vi "[FPGA] Low Pass Filter Multichannel with Alpha terminal (FXP 16,5).vi"(5 "enable":bool, 7 "Channel #":u32, 10 "LPF alpha":sgl=0.0062437057, 11 "x":sgl) -> (3 "filtered x":sgl)   [LabVIEW 2015]
uses:
  <vilib>/rvi/DataTransferAndStorage/Container/Common/niFpgaContainerGetUniqueNameForEmu.vi
  <vilib>/rvi/DataTransferAndStorage/Container/Common/niFpgaContainerSetEmuInfo.vi
  <vilib>/rvi/eio/common/nirviEmuReportErrorAndStop.vi
  <vilib>/rvi/DataTransferAndStorage/Container/Common/niFpgaContainerExecOnDevCompGetState.vi
  <vilib>/rvi/Emulation/niFpgaEmulationIsFPGAContextNoSignature.vi
  <vilib>/rvi/Emulation/niFpgaProcessEmulError.vi
  <vilib>/rvi/Emulation/niFpgaSctlEmulationGetInTimedLoop.vi
  <vilib>/rvi/errors/nirviReportUnexpectedCaseInternalError (U32).vi
  <vilib>/rvi/Memory/Memory_Emulation/niFpgaMemoryEmulationCacheClearOnFirstRun.vi
  <vilib>/rvi/Memory/Memory_Emulation/nirvimemoryEmulationManagerCache_MakeExclusive.vi
  <vilib>/rvi/Memory/Memory_Emulation/niFpgaMemoryEmulationValidateCache.vi
  <vilib>/rvi/Memory/Memory_Emulation/nirvimemoryEmulationManagerCache_InsertValue.vi
  <vilib>/Utility/error.llb/Clear Errors.vi
  <vilib>/rvi/Memory/Memory_Emulation/nirvimemoryEmulationManagerCache_ReleaseExclusive.vi
  <vilib>/rvi/Memory/Memory_Emulation/nirvimemoryEmulationManagerCache_GetValue.vi
  <vilib>/rvi/Memory/Memory_Emulation/nirvimemoryEmulationManagerCache_SetValue.vi
  <vilib>/rvi/Emulation/niFpgaSctlEmulationResourceMgr.vi
  <vilib>/rvi/LocalResourceManager/LocalResourceManager.xnode
  <vilib>/rvi/DataTransferAndStorage/Container/XNode/niFpgaContainer.xnode
  <vilib>/rvi/Memory/Memory_Emulation/niFpgaMemoryEmulationRefIn.vi
panel:
  # "= 1-1/(2*dT*fc*pi+1)"
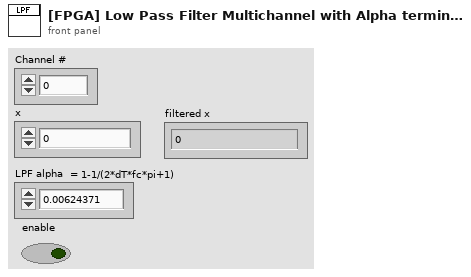
[diagram p1: front panel]
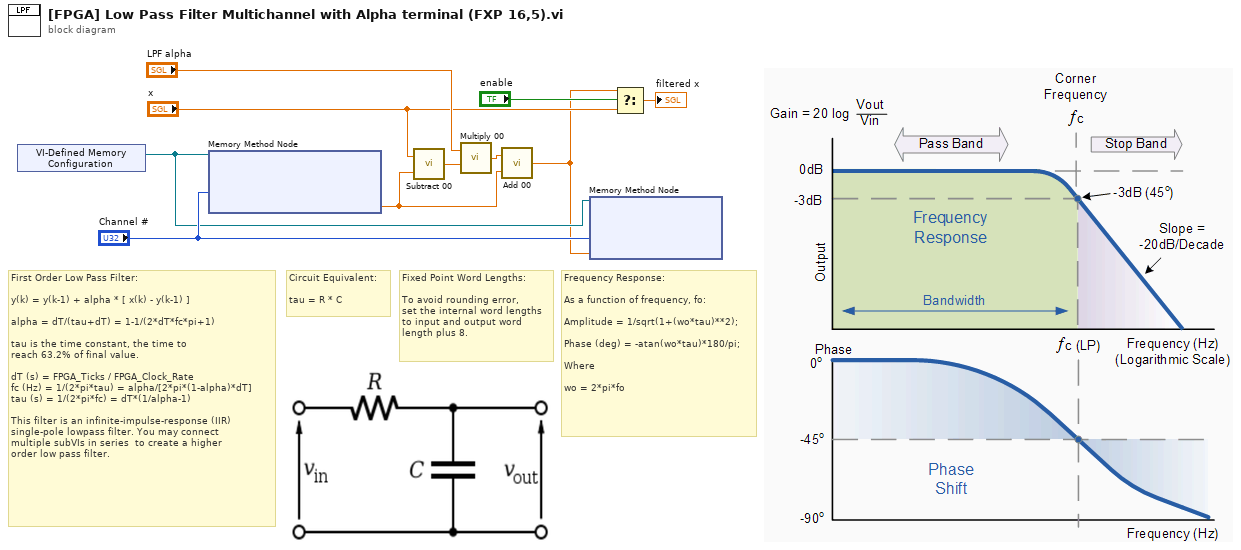
[diagram p0: block diagram]
diagram:
  # "First Order Low Pass Filter:\n\ny(k) = y(k-1) + alpha * [ x(k) - y(k-1) ]\n\nalpha = dT/(tau+dT) = 1-1/(2*dT*fc*pi+1)\n\ntau is the time constant, the time to \nreach 63.2% of final value.\n\ndT (s) = FPGA_Ticks / FPGA_Clock_Rate\nfc (Hz) = 1/(2*pi*tau) = alpha/[2*pi*(1-alpha)*dT] \ntau (s) = 1/(2*pi*fc) = dT*(1/alpha-1)\n\nThis filter is an infinite-impulse-response (IIR)\nsingle-pole lowpass filter. You may connect \nmultiple subVIs in series  to create a higher \norder low pass filter."
  # "Fixed Point Word Lengths:\n\nTo avoid rounding error,\nset the internal word lengths\nto input and output word\nlength plus 8."
  # "Frequency Response:\n\nAs a function of frequency, fo: \n\nAmplitude = 1/sqrt(1+(wo*tau)**2);\n\nPhase (deg) = -atan(wo*tau)*180/pi;\n\nWhere\n\nwo = 2*pi*fo"
  # "Circuit Equivalent:\n\ntau = R * C"
  n1 = xnode ("VI-Defined Memory Configuration")() -> ("Memory Out"=w7:refnum<k21>)
  n2 = xnode ("Memory Method Node")("Address"="Channel #", "Memory In"=w7) -> ("Data"=w6:sgl)  [unwired: 1 out]
  n3 = call "Subtract 00.vi"("y"=w6, "x"="x") -> ("x*y"=w4:sgl)
  n4 = call "Multiply 00.vi"("y"=w4, "x"="LPF alpha") -> ("x*y"=w5:sgl)
  n5 = call "Add 00.vi"("y"=w6, "x"=w5) -> ("x+y"=w1:sgl)
  n6 = xnode ("Memory Method Node")("Address"="Channel #", "Data"=w1, "Memory In"=w7) -> ()  [unwired: 1 out]
  n7 = Select(t=w1, s="enable", f="x") -> (s? t:f=→"filtered x":sgl)
